vi "measure_jv.vi"(0 "User Name":string, 1 "Cell details cluster":T2={"Cell Position"=16, "Cell Label"="", "Pixel to measure"=0, "Area (cm^2)"=0.126, "Variable"="", "Variable value"="", "Scan settings in queue"=0, "Light or dark"="", "Measurement type"=""} {"Pixel to measure" items=["All", "1", "2", "3", "4", "5", "6", "7", "8"]}, 3 "Date array":string[](array[string]), 5 "Experiment Title":string, 9 "Intensity (no. of suns)":string, 12 "Scan settings":T1={"J-V scan"=TRUE, "Start voltage (V)"=0.0, "End voltage (V)"=0.0, "Step voltage (V)"=1.4, "Scan both directions"=TRUE, "Inverted device structure"=FALSE, "Measurement delay (s)"=10.0, "Measurement speed"=0, "Scan rate (V/s)"=0.0, "Stabilisation time (s)"=0.0, "Stabilisation mode"=0, "Stabilisation value (V or A) "=1.0, "Illumination"=0, "Stabilisation in the dark?"=FALSE, "Repeat light scans"=FALSE, "No. of repeat scans"=0.0, "Only repeat for best pixel"=1, "J-t scan"=FALSE, "J-t best pixel only"=7, "J-t start voltage (V)"=0.0, "J-t end voltage (V)"=1.4, "J-t step voltage (V)"=0.01, "Step time (s)"=0.7, "J-t scan both directions"=TRUE, "J-t inverted device structure"=FALSE, "Settling delay (s)"=0.0, "J-t measurement speed"=0, "J-t illumination"=2, "Max. power stabilisation"=FALSE, "Max power best pixel only"=1, "Max. power point tracker"=FALSE, "Vmp from J-V scan"=FALSE, "Max P stab. Specific voltage"=FALSE, "Vmp (V)"=1.0, "Stabilisation time step (s)"=1.0, "Total stabilisation time (s)"=100.0} {"Settling delay (s)" min=0.0; "J-t illumination" items=["Light only", "Dark only", "Light then dark", "Dark then light"]; "Measurement speed" items=["Fast", "Normal", "High accuracy"]; "Illumination" items=["Light only", "Dark only", "Light then dark", "Dark then light"]; "Only repeat for best pixel" items=["only for best pixel", "for best 2 pixels", "for best 3 pixels", "for best 4 pixels", "for best 5 pixels", "for best 6 pixels", "for best 7 pixels", "for all pixels"]; "No. of repeat scans" min=1.0 step=1.0; "Max power best pixel only" items=["only the best pixel", "the best 2 pixels", "the best 3 pixels", "the best 4 pixels", "the best 5 pixels", "the best 6 pixels", "the best 7 pixels", "all pixels"]; "J-t best pixel only" items=["only the best pixel", "the best 2 pixels", "the best 3 pixels", "the best 4 pixels", "the best 5 pixels", "the best 6 pixels", "the best 7 pixels", "all pixels"]; "J-t measurement speed" items=["Fast", "Normal", "High Accuracy"]; "Stabilisation mode" items=["V", "I"]; "Measurement delay (s)" min=0.01}, 13 "VISA resource name":refnum<visa-resource-name>="GPIB1::24::INSTR", 14 "Skip pixel?":bool) -> (4 "JV Curve":cluster{"Y":dbl[], "Y":dbl[]}[](graph), 6 "File path for master log":path, 15 "Log Table":string[][](table))   [LabVIEW 2016]
uses:
  TypeDefs/scan_settings.ctl
  <vilib>/Utility/file.llb/Read Delimited Spreadsheet (DBL).vi
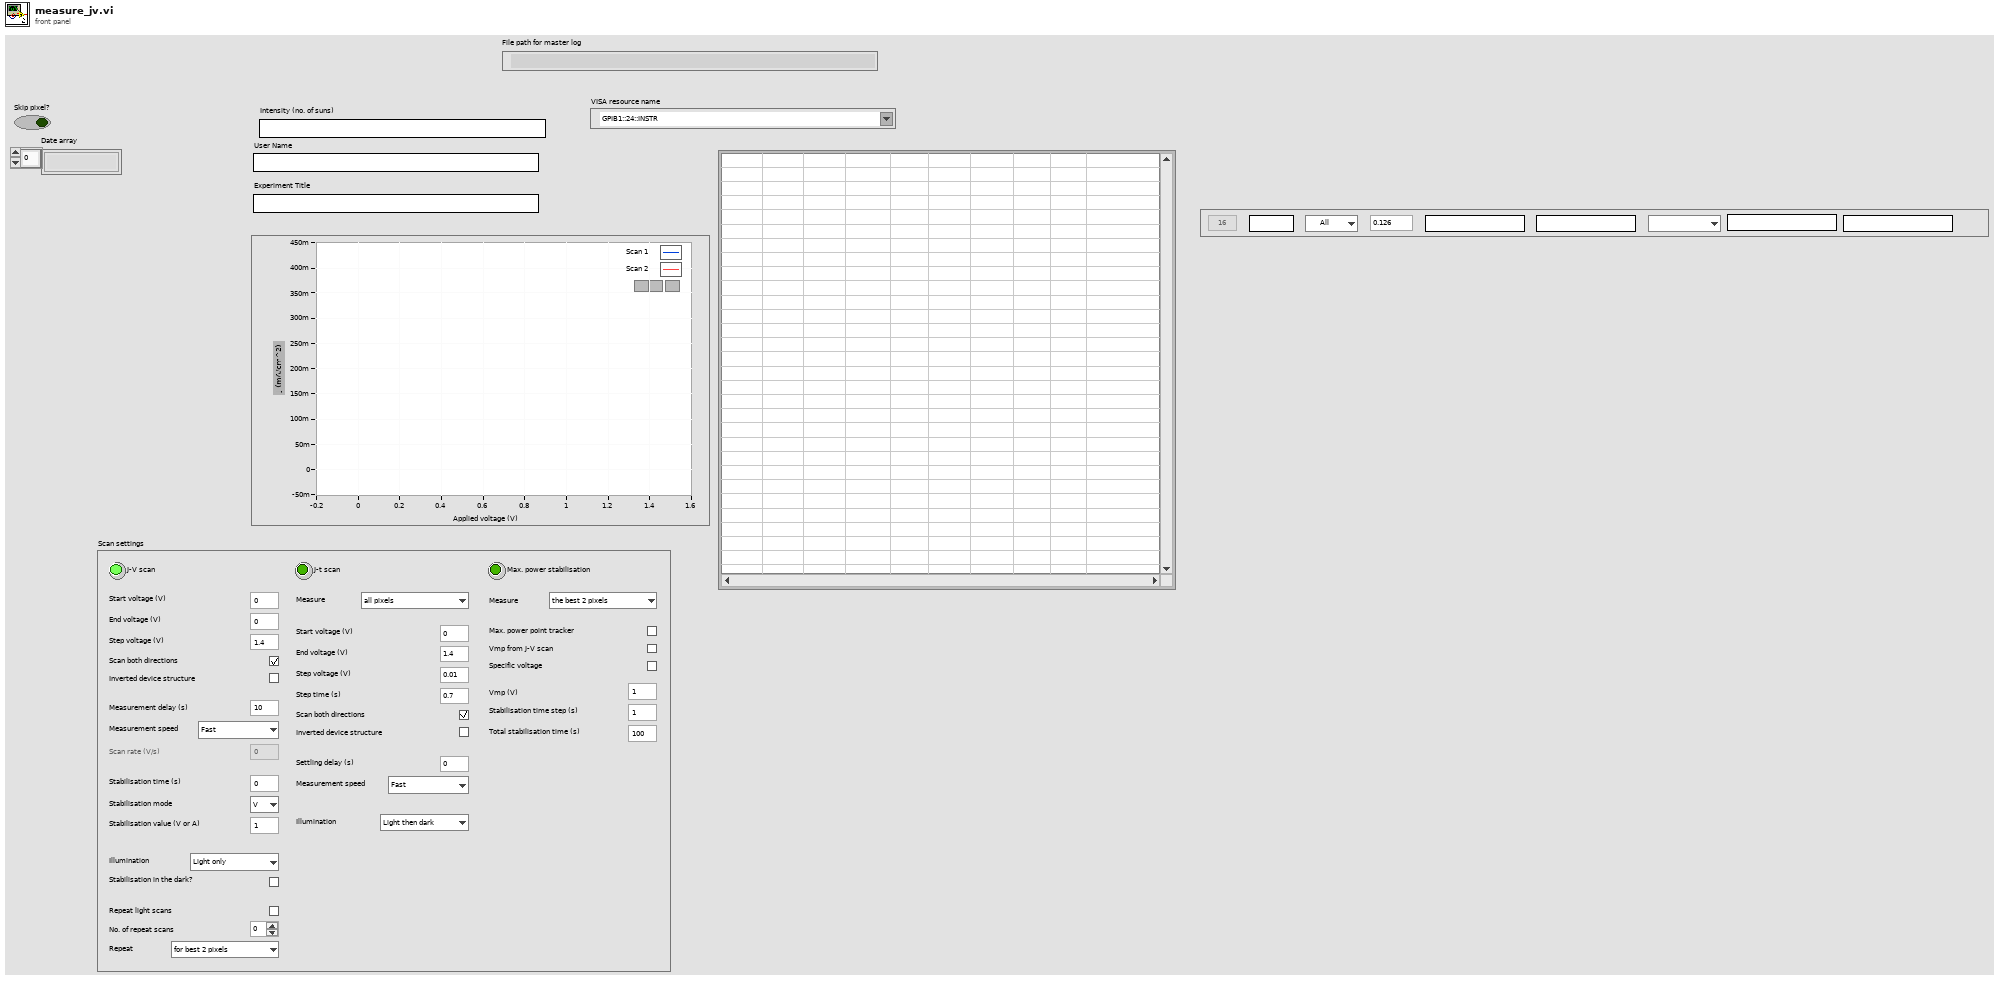
[diagram p1: front panel]
types:
  T1 = typedef "scan_settings.ctl" = cluster{"J-V scan":bool, "Start voltage (V)":dbl, "End voltage (V)":dbl, "Step voltage (V)":dbl, "Scan both directions":bool, "Inverted device structure":bool, "Measurement delay (s)":dbl, "Measurement speed":u8, "Scan rate (V/s)":dbl, "Stabilisation time (s)":dbl, "Stabilisation mode":u16, "Stabilisation value (V or A) ":dbl, "Illumination":u16, "Stabilisation in the dark?":bool, "Repeat light scans":bool, "No. of repeat scans":dbl, "Only repeat for best pixel":u16, "J-t scan":bool, "J-t best pixel only":u16, "J-t start voltage (V)":dbl, "J-t end voltage (V)":dbl, "J-t step voltage (V)":dbl, "Step time (s)":dbl, "J-t scan both directions":bool, "J-t inverted device structure":bool, "Settling delay (s)":dbl, "J-t measurement speed":u16, "J-t illumination":u16, "Max. power stabilisation":bool, "Max power best pixel only":u16, "Max. power point tracker":bool, "Vmp from J-V scan":bool, "Max P stab. Specific voltage":bool, "Vmp (V)":dbl, "Stabilisation time step (s)":dbl, "Total stabilisation time (s)":dbl}
  T2 = cluster{"Cell Position":i32, "Cell Label":string, "Pixel to measure":u16, "Area (cm^2)":dbl, "Variable":string, "Variable value":string, "Scan settings in queue":u16, "Light or dark":string, "Measurement type":string}
  T3 = typedef "imagedata.ctl" = cluster{"image type":i32, "image depth":i32, "image":u8[], "mask":u8[], "colors":u32[], "Rectangle":cluster{"left":i16, "top":i16, "right":i16, "bottom":i16}}
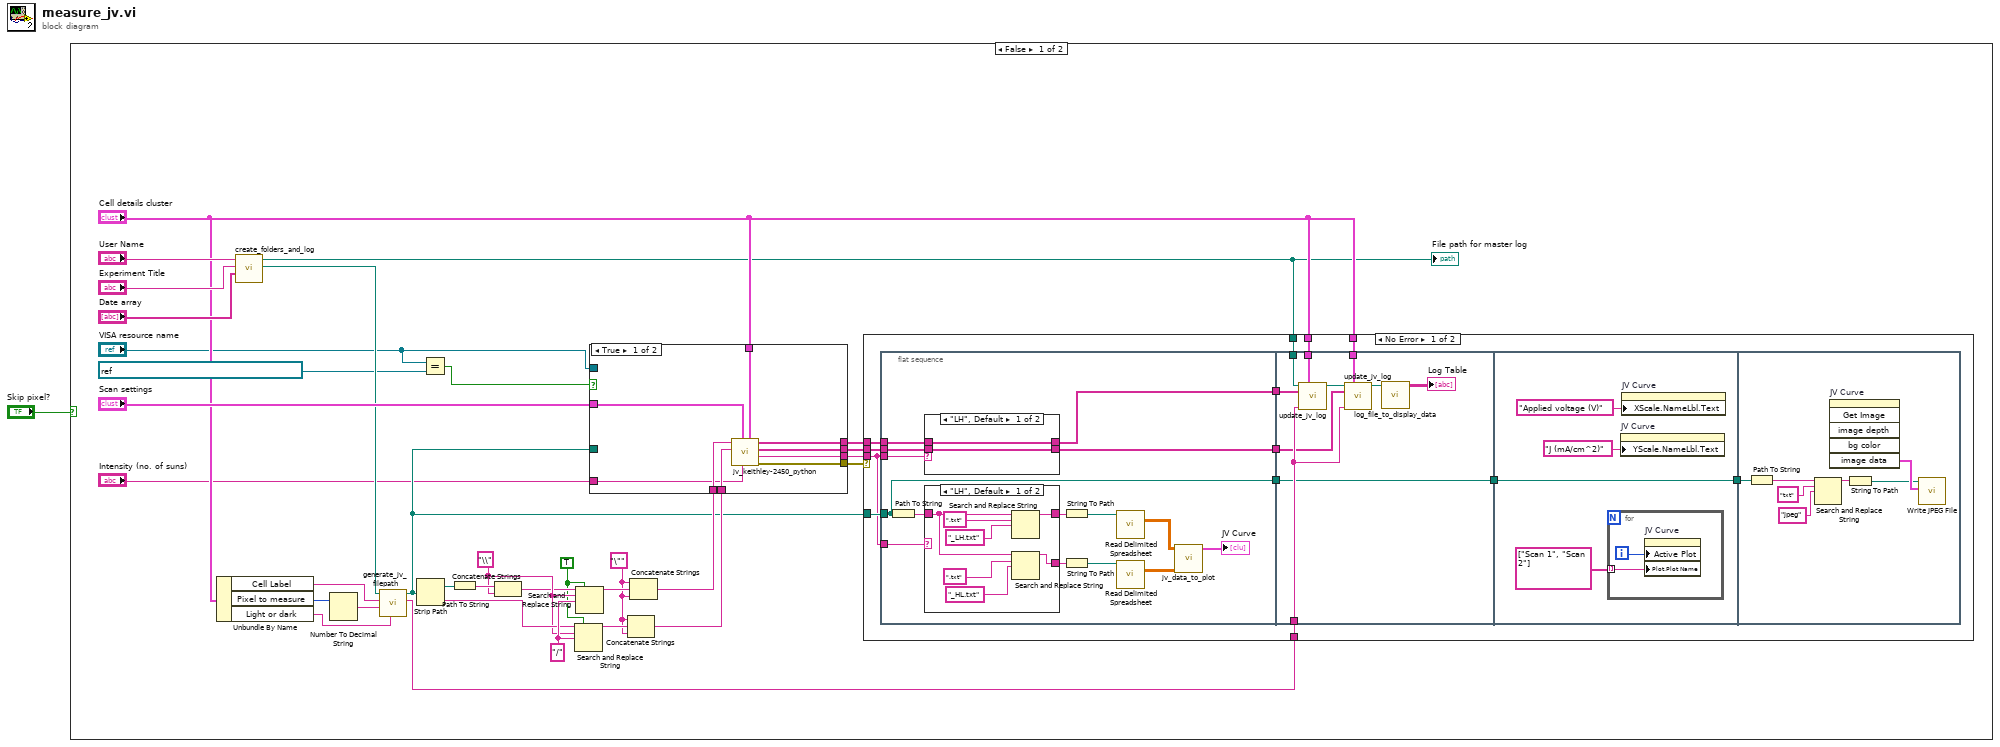
[diagram p0: block diagram]
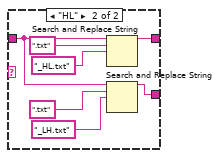
[diagram p3: hidden frame]
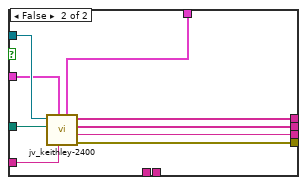
[diagram p5: hidden frame]
diagram:
  n1 = case shown="False" "Skip pixel?" {
    frame False {
      w19 = "\"" ("string")
      w16 = TRUE ("replace all? (F)")
      w24 = "/" ("search string")
      w18 = "\\" ("search string")
      n2 = Unbundle By Name("Cell details cluster") -> ("Cell Label"=w29:string, "Pixel to measure"=w30:u16, "Light or dark"=w26:string)
      n3 = call "create_folders_and_log.vi"("Date array"="Date array", "Experiment title"="Experiment Title", "Username"="User Name") -> ("Data Output Folder"=w27:path, "File path for master log"=w8:path)  [unwired: 7 in]
      "File path for master log" <- w8
      n4 = Number To Decimal String(number=w30) -> (decimal integer string=w28:string)  [unwired: 1 in]
      n5 = call "generate_jv_filepath.vi"("Light or dark"=w26, "Pixel"=w28, "Cell Label"=w29, "Data Output Folder"=w27) -> ("Scan number"=w10:string, "File path"=w12:path)  [unwired: 6 in]
      n6 = Strip Path(path=w12) -> (stripped path=w21:path, name=w22:string)
      n7 = Equal?(x="VISA resource name", y=refnum<visa-resource-name> "USB0::0x05E6::0x2450::04049675::INSTR") -> (x = y?=w3:bool)
      n8 = Path To String(path=w21) -> (string=w20:string)
      n9 = Concatenate Strings(w20, w18) -> (w17:string)
      n10 = Search and Replace String(replace all?=w16, input string=w22, search string=w18, replace string=w24) -> (result string=w23:string)  [unwired: 4 in, 3 out]
      n11 = Search and Replace String(replace all?=w16, input string=w17, search string=w18, replace string=w24) -> (result string=w25:string)  [unwired: 4 in, 3 out]
      n12 = Concatenate Strings(w19, w23, w19) -> (w14:string)
      n13 = Concatenate Strings(w19, w25, w19) -> (w15:string)
      n14 = case shown="True" w3 {
        tunnel: "VISA resource name" -> [_ w121]
        tunnel: "Scan settings" -> [w112 w120]
        tunnel: w15 -> [w111 _]
        tunnel: w14 -> [w110 _]
        tunnel: [w109 w119] -> w13
        tunnel: w12 -> [_ w118]
        tunnel: [w108 w117] -> w11
        tunnel: "Cell details cluster" -> [w107 w116]
        tunnel: [w106 w114] -> w7
        tunnel: [w105 w115] -> w6
        tunnel: "Intensity (no. of suns)" -> [w104 w113]
        frame True {
          n15 = call "jv_keithley-2450_python.vi"("Cell details cluster"=w107, "intensity (# of suns)"=w104, "Scan settings"=w112, "file name"=w110, "folder path"=w111) -> ("error out"=w109:errorcluster, "1st scan direction"=w108:string, "HL j-v metrics"=w105:string[], "LH j-v metrics"=w106:string[])  [unwired: 3 in]
        }
        frame False {
          n16 = call "jv_keithley-2400.vi"("Cell details cluster"=w116, "intensity (no. of suns)"=w113, "Scan settings"=w120, "File path for jv data"=w118, "VISA Refnum in"=w121) -> ("error out"=w119:errorcluster, "1st scan direction"=w117:string, "HL jv metrics"=w115:string[], "LH jv metrics"=w114:string[])  [unwired: 3 in]
        }
      }
      n17 = case shown="No Error" w13 {
        tunnel: w12 -> [w47 _]
        tunnel: w11 -> [w42 _]
        tunnel: w8 -> [w46 _]
        tunnel: "Cell details cluster" -> [w45 _]
        tunnel: w10 -> [w44 _]
        tunnel: "Cell details cluster" -> [w43 _]
        tunnel: w7 -> [w41 _]
        tunnel: w6 -> [w39 _]
        frame No Error {
          n18 = flat-sequence {
            tunnel: w47 -> [w48]
            tunnel: w42 -> [w54]
            tunnel: w42 -> [w53]
            tunnel: w41 -> [w52]
            tunnel: [w51] -> w40
            tunnel: w39 -> [w50]
            tunnel: [w49] -> w38
            tunnel: [w48] -> w37
            tunnel: w46 -> [w90]
            tunnel: w45 -> [w89]
            tunnel: w44 -> [w87]
            tunnel: w43 -> [w86]
            tunnel: w40 -> [w83]
            tunnel: w38 -> [w82]
            tunnel: w37 -> [w81]
            tunnel: [w81] -> w36
            tunnel: w36 -> [w91]
            tunnel: [w91] -> w35
            tunnel: w35 -> [w98]
            frame #0 {
              n19 = Path To String(path=w48) -> (string=w58:string)
              n20 = case shown="\"LH\", Default" w53 {
                tunnel: [w64 w65] -> w51
                tunnel: w52 -> [w64 w66]
                tunnel: w50 -> [w63 w65]
                tunnel: [w63 w66] -> w49
                frame "LH", Default {
                }
                frame "HL" {
                }
              }
              n21 = case shown="\"LH\", Default" w54 {
                tunnel: [w73 w80] -> w59
                tunnel: w58 -> [w68 w75]
                tunnel: [w67 w74] -> w55
                frame "LH", Default {
                  n22 = Search and Replace String(input string=w68, search string=".txt", replace string="_LH.txt" ("replace string (\"\")")) -> (result string=w67:string)  [unwired: 5 in, 3 out]
                  n23 = Search and Replace String(input string=w68, search string=".txt", replace string="_HL.txt" ("replace string (\"\")")) -> (result string=w73:string)  [unwired: 5 in, 3 out]
                }
                frame "HL" {
                  n24 = Search and Replace String(input string=w75, search string=".txt", replace string="_HL.txt" ("replace string (\"\")")) -> (result string=w74:string)  [unwired: 5 in, 3 out]
                  n25 = Search and Replace String(input string=w75, search string=".txt", replace string="_LH.txt" ("replace string (\"\")")) -> (result string=w80:string)  [unwired: 5 in, 3 out]
                }
              }
              n26 = String To Path(string=w55) -> (path=w56:path)
              n27 = String To Path(string=w59) -> (path=w60:path)
              n28 = call-poly <vilib>:"Read Delimited Spreadsheet.vi"("file path (dialog if empty)"=w56) -> ("all rows"=w57:dbl[][])  [unwired: 9 in, 5 out]
              n29 = call-poly <vilib>:"Read Delimited Spreadsheet.vi"("file path (dialog if empty)"=w60) -> ("all rows"=w61:dbl[][])  [unwired: 9 in, 5 out]
              n30 = call "jv_data_to_plot.vi"("Data Array 2"=w61, "Data Array"=w57) -> ("JV Curve"=→"JV Curve":cluster{"Y":dbl[], "Y":dbl[]}[])  [unwired: 9 in]
            }
            frame #1 {
              n31 = call "update_jv_log.vi"("File path for master log"=w90, "Cell details cluster"=w89, "j-v metrics"=w83, "scan number"=w87) -> ("File path for master log"=w88:path)  [unwired: 11 in]
              n32 = call "update_jv_log.vi"("File path for master log"=w88, "Cell details cluster"=w86, "j-v metrics"=w82, "scan number"=w87) -> ("File path for master log"=w84:path)  [unwired: 11 in]
              n33 = call "log_file_to_display_data.vi"("File path for master log"=w84) -> ("Formatted table"=→"Log Table":string[][])  [unwired: 10 in]
            }
            frame #2 {
              n34 = for {
                tunnel: string[] ["Scan 1", "Scan 2"] ("Measurement queue") -> [w95] mode=indexing
                i -> [w96]
                n35 = property on="JV Curve" class="XYGraph (strict)"("Active Plot"=w96, "Plot.Plot Name"=w95) -> ()  [unwired: 2 in, 2 out]
              }
              n36 = property on="JV Curve" class="XYGraph (strict)"("YScale.NameLbl.Text"="J (mA/cm^2)" ("Y Scale.Name Label.Text")) -> ()  [unwired: 2 in, 2 out]
              n37 = property on="JV Curve" class="XYGraph (strict)"("XScale.NameLbl.Text"="Applied voltage (V)" ("X Scale.Name Label.Text")) -> ()  [unwired: 2 in, 2 out]
            }
            frame #3 {
              n38 = Path To String(path=w98) -> (string=w102:string)
              n39 = Search and Replace String(input string=w102, search string="txt", replace string="jpeg") -> (result string=w99:string)  [unwired: 5 in, 3 out]
              n40 = invoke on="JV Curve" class="XYGraph (strict)" method="Get Image"() -> ("image data"=w103:T3)  [unwired: 6 in, 5 out]
              n41 = String To Path(string=w99) -> (path=w97:path)
              n42 = call <vilib>:"Write JPEG File.vi"("image data"=w103, "path to JPEG file"=w97) -> ()  [unwired: 8 in, 2 out]
            }
          }
        }
        frame Error {
        }
      }
    }
    frame True {
    }
  }
